vi "Load_VI_Icon_Parts.vi"(8 "error in (no error)":errorcluster, 10 "VI Refnum":refnum<vi>, 11 "AB_SourceDistribution in":refnum<class "AB_PackedLibrary.lvclass">) -> (0 "error out":errorcluster, 2 "VI Refnum Out":refnum<vi>, 3 "AB_SourceDistribution out":refnum<class "AB_PackedLibrary.lvclass">)   [LabVIEW 2020, in "AB_PackedLibrary.lvclass"]
uses:
  <vilib>/AppBuilder/AB_Classes/PackedLib/AB_PackedLibrary.lvclass
  <vilib>/picture/picture.llb/imagedata.ctl
  <vilib>/AppBuilder/AB_Classes/TargetFile/AB_Targetfile.lvclass
panel:
  out "Color 256":T1
  out "Color 16":T1
  out "Monochrome":T1
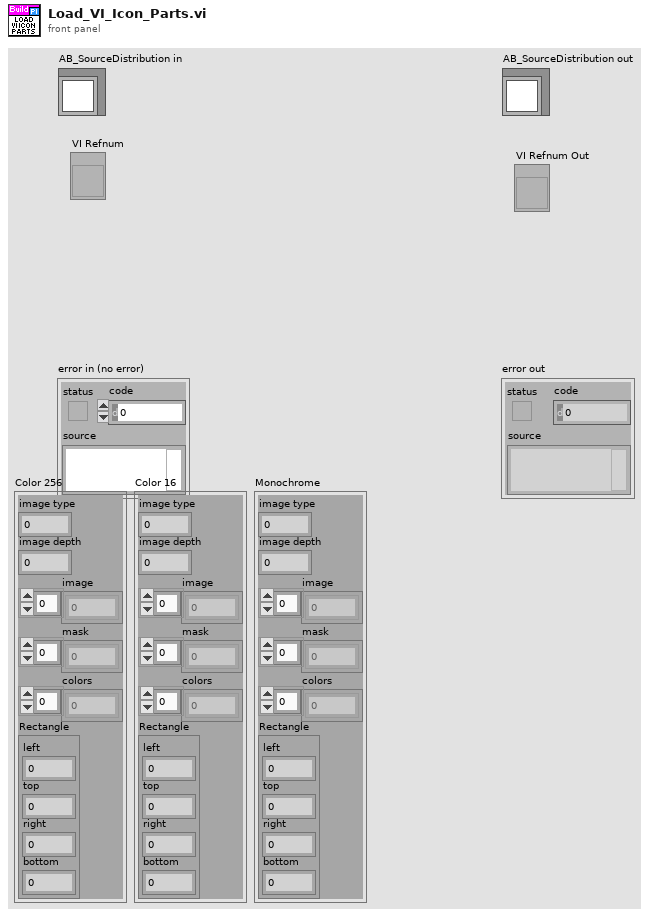
[diagram p1: front panel]
types:
  T1 = typedef "imagedata.ctl" = cluster{"image type":i32, "image depth":i32, "image":u8[], "mask":u8[], "colors":u32[], "Rectangle":cluster{"left":i16, "top":i16, "right":i16, "bottom":i16}}
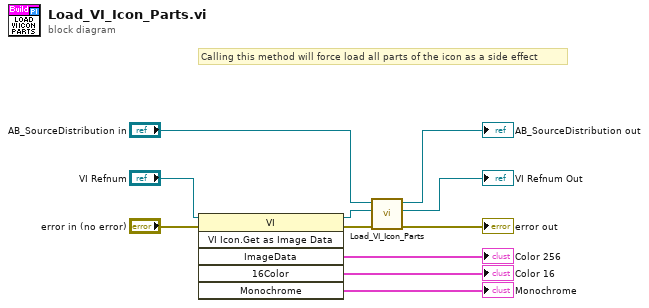
[diagram p0: block diagram]
diagram:
  # "Calling this method will force load all parts of the icon as a side effect"
  n1 = invoke class="VI" method="VI Icon.Get as Image Data"(reference="VI Refnum", error in="error in (no error)") -> (reference out=w7:refnum<vi>, error out=w1:errorcluster, "ImageData"=→"Color 256":T1, "16Color"=→"Color 16":T1, "Monochrome"=→"Monochrome":T1)  [unwired: 4 in, 1 out]
  n2 = call-parent "Load_VI_Icon_Parts.vi"("error in (no error)"=w1, "VI Refnum"=w7, "AB_Build in"="AB_SourceDistribution in") -> ("error out"=→"error out":errorcluster, "VI Refnum Out"=→"VI Refnum Out":refnum<vi>, "AB_Build out"=→"AB_SourceDistribution out":refnum<class "AB_PackedLibrary.lvclass">)  [unwired: 6 in]
